vi "Configure Data Log Trigger.vi"(6 "Data Log Trigger Slope (1: Positive)":u16(ring)=1 items=["Negative", "Positive"], 7 "Data Log Trigger Level (0.0)":dbl format="%^.3e", 8 "error in (no error)":errorcluster {"code" format="%.0x"}, 9 "Data Log Type (1: Voltage)":i32(ring)=1 items=["Voltage"=1, "Current"=0], 10 "Channel Name (1)":string="1", 11 "VISA resource name":refnum<visa-resource-name>) -> (0 "error out":errorcluster {"code" format="%.0x"}, 3 "VISA resource name out":refnum<visa-resource-name>)   [LabVIEW 2014, in "Agilent N6700 Series.lvlib"]
doc: "Configures the trigger for the data logger.\n\n<b>Note:</b>\nThis VI only applies to the N6705B and N6705C DC Power Analyzer."
uses:
  Agilent N6700 Series.lvlib
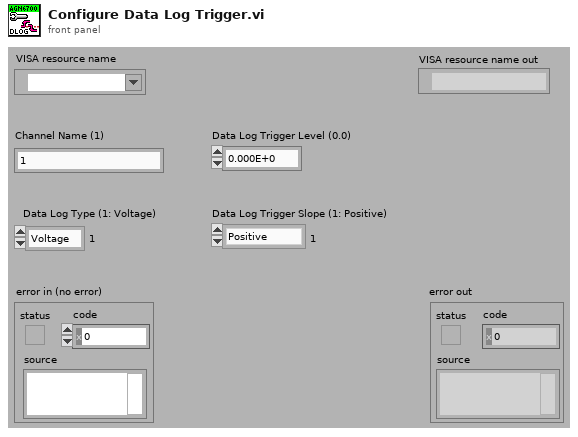
[diagram p1: front panel]
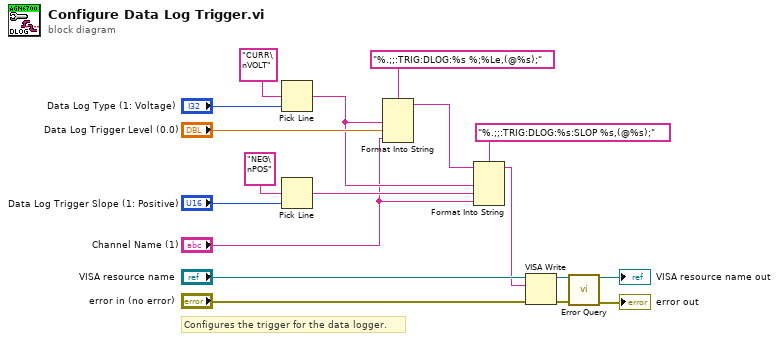
[diagram p0: block diagram]
diagram:
  # "Configures the trigger for the data logger."
  n1 = Pick Line(multi-line string="CURR\nVOLT", line index="Data Log Type (1: Voltage)") -> (output string=w3:string)  [unwired: 1 in]
  n2 = Pick Line(multi-line string="NEG\nPOS", line index="Data Log Trigger Slope (1: Positive)") -> (output string=w4:string)  [unwired: 1 in]
  n3 = Format Into String(format string="%.;;:TRIG:DLOG:%s %;%Le,(@%s);", w3, "Data Log Trigger Level (0.0)", "Channel Name (1)") -> (resulting string=w12:string)  [unwired: 2 in, 1 out]
  n4 = Format Into String(format string="%.;;:TRIG:DLOG:%s:SLOP %s,(@%s);", initial string=w12, w3, w4, "Channel Name (1)") -> (resulting string=w1:string)  [unwired: 1 in, 1 out]
  n5 = VISA Write(VISA resource name="VISA resource name", write buffer=w1, error in (no error)="error in (no error)") -> (VISA resource name out=w14:refnum<visa-resource-name>, error out=w13:errorcluster)  [unwired: 1 out]
  n6 = call "Error Query.vi"("VISA resource name"=w14, "error in (no error)"=w13) -> ("VISA resource name out"=→"VISA resource name out":refnum<visa-resource-name>, "error out"=→"error out":errorcluster)  [unwired: 10 in, 2 out]
